vi "scan harm(SubVI).vi"(10 "输出数组":string[][](array[string]), 11 "Numeric":i32) -> (2 "Array 2":dbl[](array[numeric]), 3 "Array":dbl[](array[numeric]))   [LabVIEW 2019]
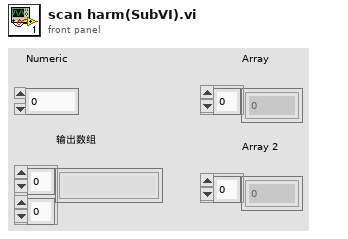
[diagram p1: front panel]
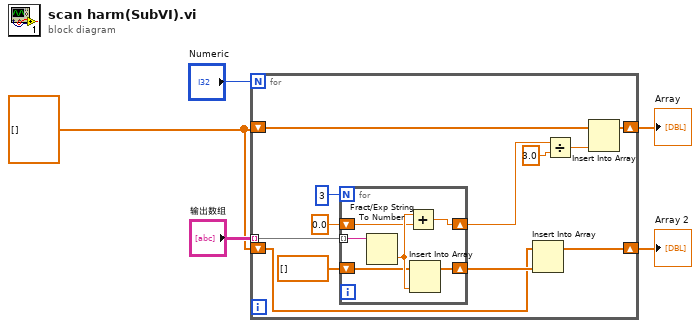
[diagram p0: block diagram]
diagram:
  w1 = dbl[] []
  n1 = for {
    N: "Numeric" -> [_]
    tunnel: "输出数组" -> [w16] mode=indexing
    shift-right: [w17] -> w3
    shift-left: w1 -> [w6]
    shift-right: [w11] -> w5
    shift-left: w1 -> [w7]
    n2 = for {
      N: 3 -> [_]
      tunnel: w16 -> [w23] mode=indexing
      shift-right: [w21] -> w15
      shift-left: dbl[] [] -> [w20]
      shift-right: [w19] -> w14
      shift-left: 0.0 -> [w18]
      n3 = Fract/Exp String To Number(string=w23) -> (number=w22:dbl)  [unwired: 3 in, 1 out]
      n4 = Add(x=w22, y=w18) -> (x+y=w19:dbl)
      n5 = Insert Into Array(array=w20, new element=w22) -> (w21:dbl[])  [unwired: 1 in]
    }
    n6 = Insert Into Array(array=w6, new element=w15) -> (w17:dbl[])  [unwired: 1 in]
    n7 = Divide(x=w14, y=3.0) -> (x/y=w12:dbl)
    n8 = Insert Into Array(array=w7, new element=w12) -> (w11:dbl[])  [unwired: 1 in]
  }
  "Array" <- w5
  "Array 2" <- w3
